vi "CRC.vi"(1 "Data In[]":u8[](array[numeric]) format="%.0x") -> (0 "CRC Out":u16 format="%.0x")   [LabVIEW 2020, in "Plugin Instrument Driver.lvlib" / "VISA Interface.lvclass"]
doc: "Calculates 16 bit CRC Value for the input byte array."
uses:
  VISA Interface.lvclass
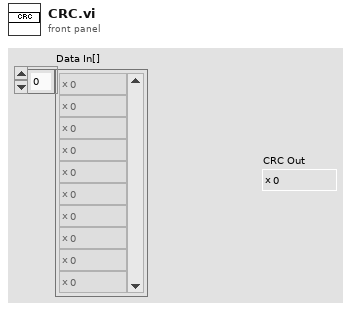
[diagram p1: front panel]
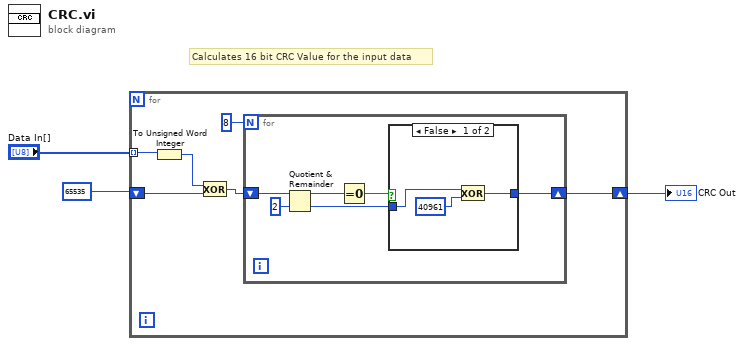
[diagram p0: block diagram]
diagram:
  # "Calculates 16 bit CRC Value for the input data"
  n1 = for {
    tunnel: "Data In[]" -> [w9] mode=indexing
    shift-right: [w4] -> w3
    shift-left: u16 65535 ("CRC") -> [w7]
    n2 = To Unsigned Word Integer(number=w9) -> (unsigned 16bit integer=w8:u16)
    n3 = Exclusive Or(1:w7, 2:w8) -> (0:w5:u16)
    n4 = for {
      N: 8 -> [_]
      shift-right: [w10] -> w4
      shift-left: w5 -> [w15]
      n5 = Quotient & Remainder(x=w15, y=u16 2) -> (x-y*floor(x/y)=w13:u16, floor(x/y)=w11:u16)
      n6 = Equal To 0?(x=w13) -> (x = 0?=w12:bool)
      n7 = case shown="False" w12 {
        tunnel: w11 -> [w18 w19]
        tunnel: [w16 w19] -> w10
        frame False {
          n8 = Exclusive Or(1:u16 40961 ("y"), 2:w18) -> (0:w16:u16)
        }
        frame True {
        }
      }
    }
  }
  "CRC Out" <- w3
